vi "Remove Frames From Port Dialog.vi"(8 "error in":errorcluster, 11 "Port Ref":T1 format="%.0x") -> (0 "error out":errorcluster, 3 "Port Ref out":T1 format="%.0x")   [LabVIEW 2020, in "Communication Bus Template System Explorer.lvlib" / "Implementation.lvlib"]
uses:
  Implementation.lvlib
  <vilib>/NI VeriStand/Custom Device API/Custom Device Item Ref.ctl
  Scripting/Constants.vi
  <vilib>/NI VeriStand/Custom Device API/Custom Device API.lvlib
  Scripting/Communication Bus Template Scripting.lvlib
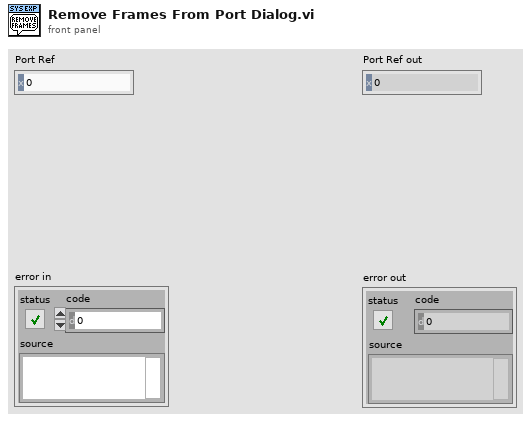
[diagram p1: front panel]
types:
  T1 = typedef "Custom Device API.lvlib/Custom Device Item Ref.ctl" = u64
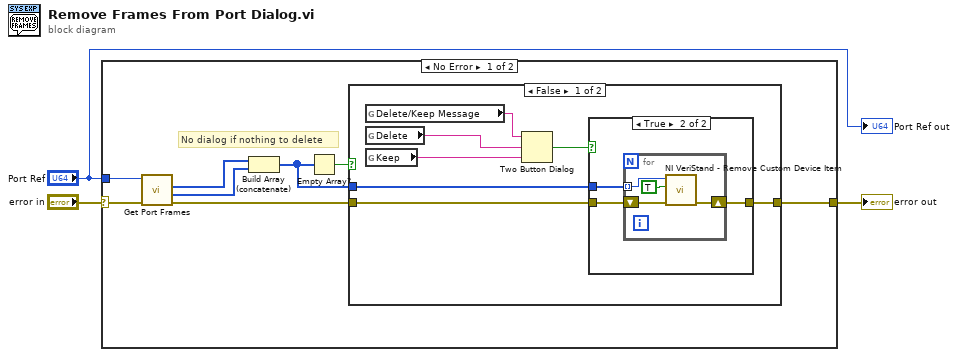
[diagram p0: block diagram]
diagram:
  n1 = case shown="No Error" "error in" {
    selector: "error in" -> [w8 w28]
    tunnel: [w11 w28] -> w2
    tunnel: "Port Ref" -> [w7 _]
    frame No Error {
      # "No dialog if nothing to delete"
      n2 = call "Get Port Frames.vi"("error in"=w8, "Port Ref"=w7) -> ("error out"=w4:errorcluster, "Outgoing Frames"=w5:T1[], "Incoming Frames"=w6:T1[])  [unwired: 6 in, 1 out]
      n3 = Build Array (concatenate)(w6, w5) -> (w10:T1[])
      n4 = Empty Array?(array=w10) -> (empty?=w9:bool)
      n5 = case shown="False" w9 {
        tunnel: w4 -> [w16 w27]
        tunnel: [w18 w27] -> w11
        tunnel: w10 -> [w17 _]
        frame False {
          n6 = global read "Constants.vi" "Delete/Keep Message"() -> (w13:string)
          n7 = global read "Constants.vi" "Delete"() -> (w15:string)
          n8 = global read "Constants.vi" "Keep"() -> (w14:string)
          n9 = Two Button Dialog(message=w13, 1:w14, 2:w15) -> (T button?=w12:bool)
          n10 = case shown="True" w12 {
            tunnel: [w19 w22] -> w18
            tunnel: w17 -> [_ w21]
            tunnel: w16 -> [w19 w20]
            frame False {
            }
            frame True {
              n11 = for {
                tunnel: w21 -> [w26] mode=indexing
                shift-right: [w24] -> w22
                shift-left: w20 -> [w25]
                n12 = call <vilib>:"NI VeriStand - Remove Custom Device Item.vi"("error in (no error)"=w25, "Force Delete (F)"=TRUE, "Item Ref in"=w26) -> ("error out"=w24:errorcluster)  [unwired: 7 in, 1 out]
              }
            }
          }
        }
        frame True {
        }
      }
    }
    frame Error {
    }
  }
  "error out" <- w2
  "Port Ref out" <- "Port Ref"
